vi "publish in mapping.vi"(7 "module ID":string, 8 "error in":errorcluster, 10 "published element":string, 11 "mappings in":T1) -> (0 "error out":errorcluster, 3 "mappings out":T1)   [LabVIEW 2013, in "engine configuration.lvclass"]
uses:
  engine configuration.lvclass
  simple mapping.ctl
  module channel pairings.ctl
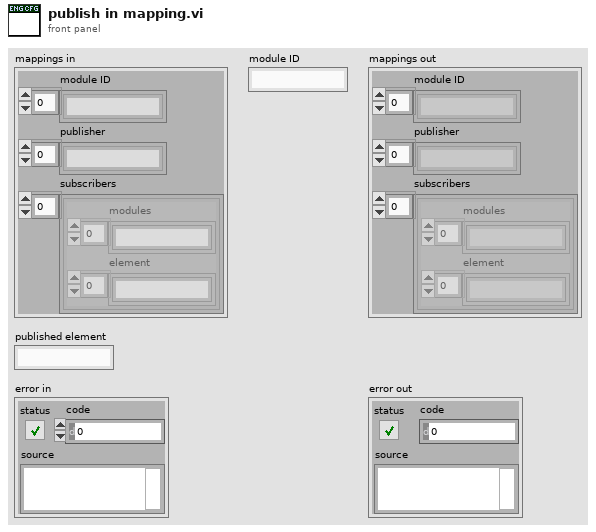
[diagram p1: front panel]
types:
  T1 = typedef "engine configuration.lvclass/simple mapping.ctl" = cluster{"module ID":string[], "publisher":string[], "subscribers":T2[]}
  T2 = typedef "engine configuration.lvclass/module channel pairings.ctl" = cluster{"modules":string[], "element":string[]}
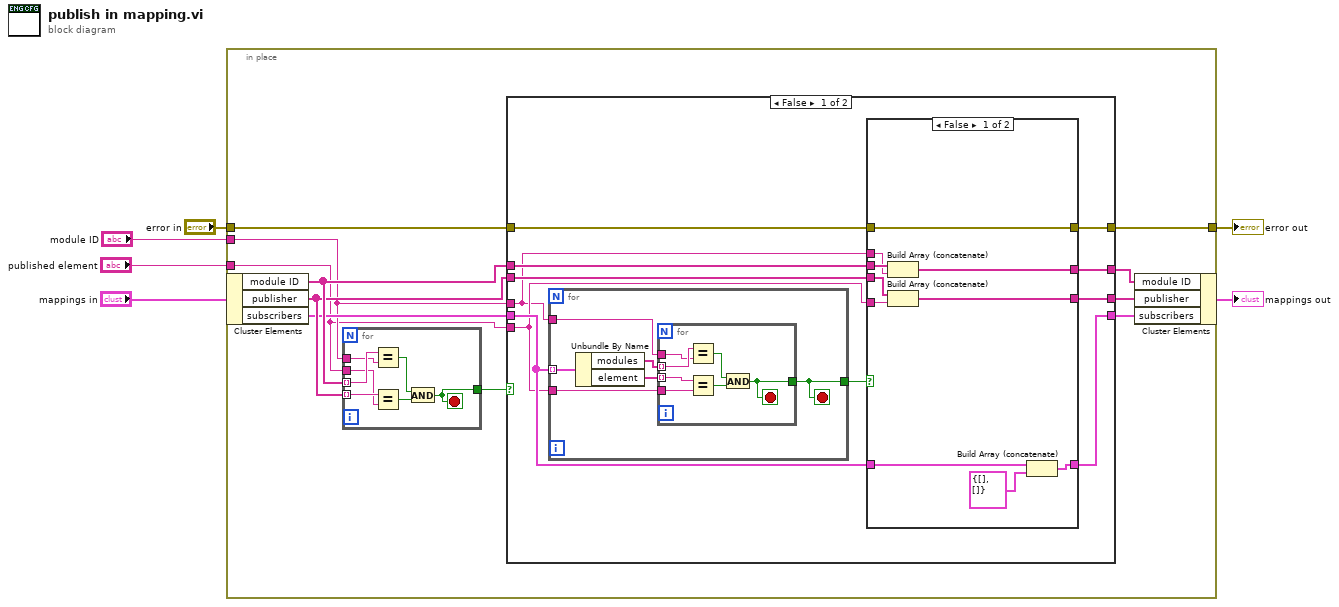
[diagram p0: block diagram]
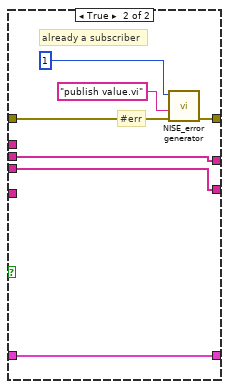
[diagram p2: hidden frame]
diagram:
  n1 = in-place {
    in-place-border: "module ID" -> [w8]
    in-place-border: "published element" -> [w7]
    in-place-border: [w10] -> w5
    in-place-border: "error in" -> [w9]
    n2 = in-place-cluster #1("mappings in") -> ("module ID"=w15:string[], "publisher"=w14:string[], "subscribers"=w11:T2[])
    n3 = for {
      tunnel: w15 -> [w69] mode=indexing
      tunnel: w14 -> [w68] mode=indexing
      tunnel: w8 -> [w67]
      tunnel: w7 -> [w66]
      tunnel: [w63] -> w17
      stop <- w63 stop-if-true
      n4 = Equal?(x=w69, y=w67) -> (x = y?=w64:bool)
      n5 = Equal?(x=w68, y=w66) -> (x = y?=w65:bool)
      n6 = And(x=w64, y=w65) -> (x .and. y?=w63:bool)
    }
    n7 = case shown="False" w17 {
      tunnel: [w21 w62] -> w16
      tunnel: w15 -> [w20 w62]
      tunnel: w14 -> [w23 w61]
      tunnel: [w22 w61] -> w13
      tunnel: [w25 w60] -> w12
      tunnel: w11 -> [w24 w60]
      tunnel: [w27 w59] -> w10
      tunnel: w9 -> [w26 w59]
      tunnel: w7 -> [w19 _]
      tunnel: w8 -> [w18 _]
      frame False {
        n8 = for {
          tunnel: w24 -> [w51] mode=indexing
          tunnel: [w48] -> w28
          tunnel: w18 -> [w47]
          tunnel: w19 -> [w46]
          stop <- w48 stop-if-true
          n9 = Unbundle By Name(w51) -> ("modules"=w50:string[], "element"=w49:string[])
          n10 = for {
            tunnel: w50 -> [w56] mode=indexing
            tunnel: w49 -> [w55] mode=indexing
            tunnel: [w54] -> w48
            tunnel: w47 -> [w53]
            tunnel: w46 -> [w52]
            stop <- w54 stop-if-true
            n11 = Equal?(x=w56, y=w53) -> (x = y?=w57:bool)
            n12 = Equal?(x=w55, y=w52) -> (x = y?=w58:bool)
            n13 = And(x=w57, y=w58) -> (x .and. y?=w54:bool)
          }
        }
        n14 = case shown="False" w28 {
          tunnel: [w38 w44] -> w27
          tunnel: w26 -> [w38 w45]
          tunnel: [w32 w41] -> w25
          tunnel: w24 -> [w33 w41]
          tunnel: w23 -> [w35 w40]
          tunnel: [w34 w40] -> w22
          tunnel: [w36 w39] -> w21
          tunnel: w20 -> [w37 w39]
          tunnel: w18 -> [w31 _]
          tunnel: w19 -> [w30 _]
          frame False {
            n15 = Build Array (concatenate)(w37, w31) -> (w36:string[])
            n16 = Build Array (concatenate)(w35, w30) -> (w34:string[])
            n17 = Build Array (concatenate)(w33, T2 {"modules"=[], "element"=[]} ("cluster of array of strings")) -> (w32:T2[])
          }
          frame True {
            # "#err"
            # "already a subscriber"
            n18 = call <vilib>:"NISE_error generator.vi"("error in"=w45, "source"="publish value.vi", "error code (0)"=1) -> ("error out"=w44:errorcluster)  [unwired: 6 in]
          }
        }
      }
      frame True {
        # "already published"
      }
    }
    n19 = in-place-cluster #1("module ID"=w16, "publisher"=w13, "subscribers"=w12) -> (→"mappings out":T1)
  }
  "error out" <- w5
